vi "read_attributes.vi"(8 "error in (no error)":errorcluster, 11 "SparsePCA in":refnum<class "SparsePCA.lvclass">) -> (0 "error out":errorcluster, 2 "attributes":T1, 3 "SparsePCA out":refnum<class "SparsePCA.lvclass">)   [LabVIEW 2020, in "SparsePCA.lvclass"]
uses:
  SparsePCA.lvclass
  Controls/sparse_pca_attributes.ctl
  SparsePCA.lvclass/SparsePCA.ctl
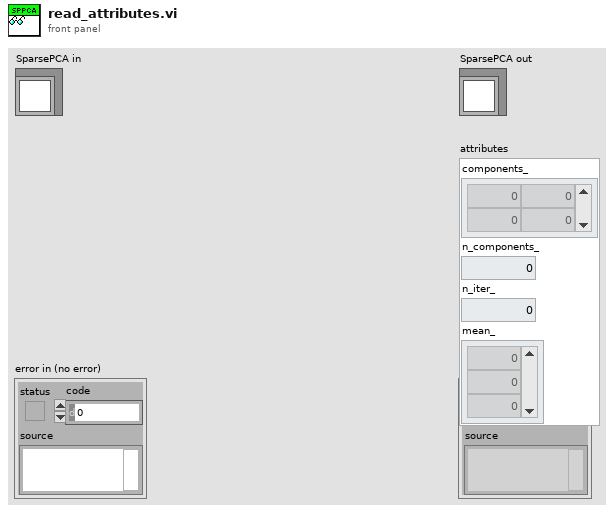
[diagram p1: front panel]
types:
  T1 = typedef "sparse_pca_attributes.ctl" = cluster{"components_":dbl[][], "n_components_":dbl, "n_iter_":dbl, "mean_":dbl[]}
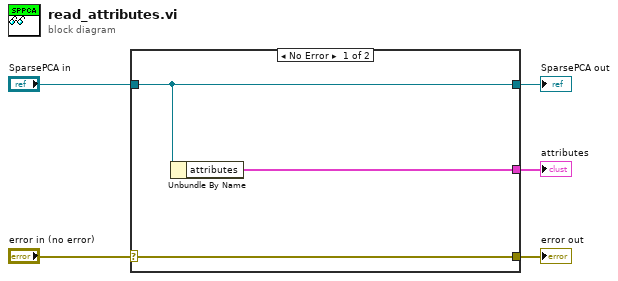
[diagram p0: block diagram]
diagram:
  n1 = case shown="No Error" "error in (no error)" {
    selector: "error in (no error)" -> [w8 w9]
    tunnel: [w8 w9] -> w4
    tunnel: [w7 w10] -> w2
    tunnel: "SparsePCA in" -> [w7 w10]
    tunnel: [w6 _] -> w1
    frame No Error {
      n2 = Unbundle By Name(w7) -> ("attributes"=w6:T1)
    }
    frame Error {
    }
  }
  "error out" <- w4
  "SparsePCA out" <- w2
  "attributes" <- w1
